vi "golpi_mpc_get_access.vi"(7 "don't query version (true)":bool=TRUE, 8 "error in":errorcluster, 10 "allow octave start (true)":bool=TRUE, 11 "golpi session ref":T1) -> (0 "error out":errorcluster, 1 "GOLPI ref out":T2={"pipe handle"={"lv_proc.dll file path"=path "", "process instance handle"=[], "debug mode"=FALSE, "debug data"=[]}, "fast read timeout [ms]"=500, "fast read settle time [ms]"=10, "fast read to multiple [ms]"=1, "max elements per input line"=100, "slow read timeout [ms]"=5000, "stdin double format specifier"="%_16e", "max elements per stdout output column"=100, "console mode bitstream"=FALSE, "bitstream first read timeout [ms]"=1000, "bitstream read timeout [ms]"=50, "struct transfer possible"=FALSE, "matlab mode"=FALSE}, 2 "golpi session out":T4={"GOLPI ref"={"pipe handle"={"lv_proc.dll file path"=path "", "process instance handle"=[], "debug mode"=FALSE, "debug data"=[]}, "fast read timeout [ms]"=500, "fast read settle time [ms]"=10, "fast read to multiple [ms]"=1, "max elements per input line"=100, "slow read timeout [ms]"=5000, "stdin double format specifier"="%_16e", "max elements per stdout output column"=100, "console mode bitstream"=FALSE, "bitstream first read timeout [ms]"=1000, "bitstream read timeout [ms]"=50, "struct transfer possible"=FALSE, "matlab mode"=FALSE}, "idn str"="", "octave path"=path "C:/Octave364/Octave3.6.4_gcc4.6.2/bin", "work path"=path "C:/Octave364/Octave3.6.4_gcc4.6.2/bin", "start timeout [ms]"=15000, "clr cache"=FALSE, "console"=FALSE, "binary"=FALSE, "semaphore"=refnum, "initial command"="", "exit command"="", "matlab"=FALSE}, 3 "golpi session ref out (copy)":T1, 4 "octave started (was closed)":bool, 5 "GNU Octave version":string)   [LabVIEW 2018, in "GOLPI Multi Process.lvlib"]
doc: "Call this to gain exclusive access to the GOLPI session (for multi-process communication). It won't return until it gets access to the GOLPI session. \n\nOptionally (by default) it will start GOLPI before returning GOLPI reference. It returns GOLPI reference - the main cluster for GOLPI library. It also returns full GOLPI session (the cluster including access semaphore and some configuarition for the mutli-process GOLPI lib). \n\nWhen work with GOLPI is done the reference must be released again by calling 'golpi_mpc_release'!"
uses:
  GOLPI Multi Process.lvlib
  golpi_session.ctl
  GOLPI Library.lvlibp/Public/GOLPI reference Type Def.ctl
  GOLPI Library.lvlibp/LV Process source distribution/Pipe Handle.ctl
  golpi_session_ref.ctl
  GOLPI Library.lvlibp/LV Process source distribution/LV Process library.lvlib
  GOLPI Library.lvlibp
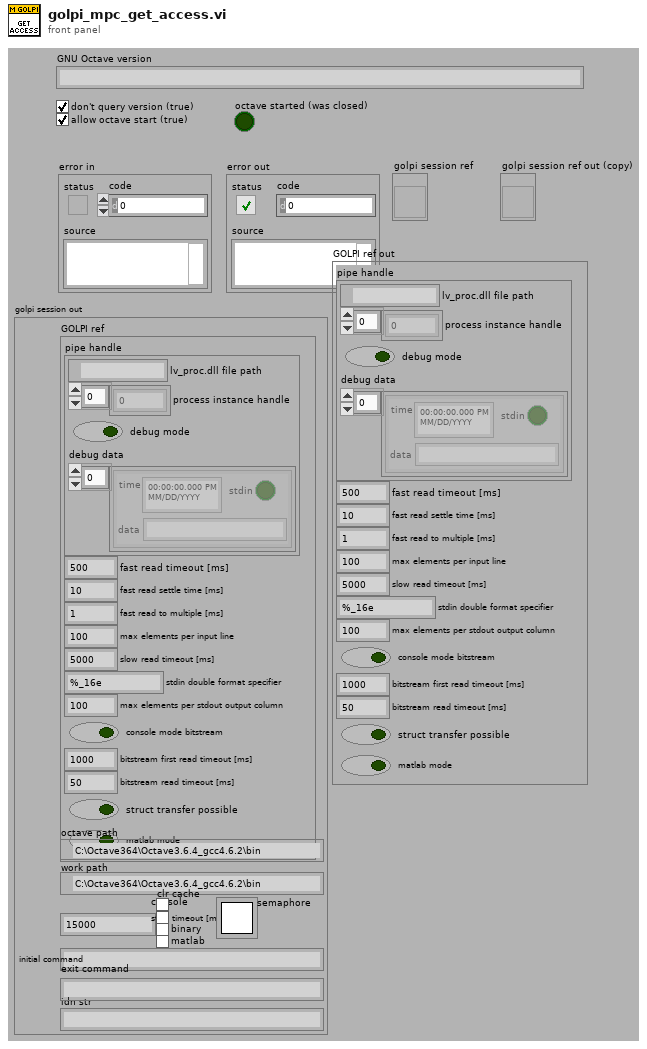
[diagram p1: front panel]
types:
  T1 = typedef "GOLPI Multi Process.lvlib/golpi_session_ref.ctl" = refnum<vi>
  T2 = typedef "GOLPI Library.lvlibp/GOLPI reference Type Def.ctl" = cluster{"pipe handle":T3, "fast read timeout [ms]":u32, "fast read settle time [ms]":u32, "fast read to multiple [ms]":u32, "max elements per input line":u32, "slow read timeout [ms]":u32, "stdin double format specifier":string, "max elements per stdout output column":u32, "console mode bitstream":bool, "bitstream first read timeout [ms]":u32, "bitstream read timeout [ms]":u32, "struct transfer possible":bool, "matlab mode":bool}
  T3 = typedef "GOLPI Library.lvlibp/LV Process library.lvlib/Pipe Handle.ctl" = cluster{"lv_proc.dll file path":path, "process instance handle":u32[], "debug mode":bool, "debug data":cluster{"time":timestamp, "stdin":bool, "data":string}[]}
  T4 = typedef "GOLPI Multi Process.lvlib/golpi_session.ctl" = cluster{"GOLPI ref":T2, "idn str":string, "octave path":path, "work path":path, "start timeout [ms]":u32, "clr cache":bool, "console":bool, "binary":bool, "semaphore":T5, "initial command":string, "exit command":string, "matlab":bool}
  T5 = typedef "Semaphore RefNum" = refnum<k1>
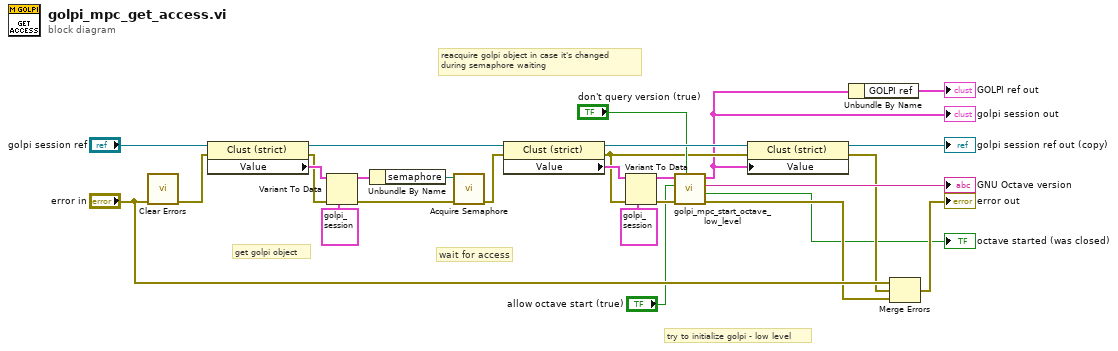
[diagram p0: block diagram]
diagram:
  # "try to initialize golpi - low level"
  # "reacquire golpi object in case it's changed\nduring semaphore waiting"
  # "wait for access"
  # "get golpi object"
  n1 = call <vilib>:"Clear Errors.vi"("error in (no error)"="error in") -> ("error out"=w12:errorcluster)  [unwired: 5 in, 1 out]
  n2 = property class="Clust (strict)"(reference="golpi session ref", error in=w12) -> (reference out=w19:T1, error out=w20:errorcluster, "Value"=w25:T4)
  n3 = Variant To Data(error in=w20, type=T4 {"GOLPI ref"={"pipe handle"={"lv_proc.dll file path"=path "", "process instance handle"=[], "debug mode"=FALSE, "debug data"=[]}, "fast read timeout [ms]"=0, "fast read settle time [ms]"=0, "fast read to multiple [ms]"=0, "max elements per input line"=0, "slow read timeout [ms]"=0, "stdin double format specifier"="", "max elements per stdout output column"=0, "console mode bitstream"=FALSE, "bitstream first read timeout [ms]"=0, "bitstream read timeout [ms]"=0, "struct transfer possible"=FALSE, "matlab mode"=FALSE}, "idn str"="", "octave path"=path "C:/Octave364/Octave3.6.4_gcc4.6.2/bin", "work path"=path "", "start timeout [ms]"=0, "clr cache"=FALSE, "console"=FALSE, "binary"=FALSE, "semaphore"=refnum, "initial command"="", "exit command"="", "matlab"=FALSE} ("golpi session"), Variant=w25) -> (data=w21:T4, error out=w23:errorcluster)
  n4 = Unbundle By Name(w21) -> ("semaphore"=w22:T5)
  n5 = call <vilib>:"Acquire Semaphore.vi"("error in (no error)"=w23, "semaphore"=w22) -> ("error out"=w16:errorcluster)  [unwired: 3 in, 2 out]
  n6 = property class="Clust (strict)"(reference=w19, error in=w16) -> (reference out=w15:T1, error out=w6:errorcluster, "Value"=w17:T4)
  n7 = Variant To Data(error in=w6, type=T4 {"GOLPI ref"={"pipe handle"={"lv_proc.dll file path"=path "", "process instance handle"=[], "debug mode"=FALSE, "debug data"=[]}, "fast read timeout [ms]"=0, "fast read settle time [ms]"=0, "fast read to multiple [ms]"=0, "max elements per input line"=0, "slow read timeout [ms]"=0, "stdin double format specifier"="", "max elements per stdout output column"=0, "console mode bitstream"=FALSE, "bitstream first read timeout [ms]"=0, "bitstream read timeout [ms]"=0, "struct transfer possible"=FALSE, "matlab mode"=FALSE}, "idn str"="", "octave path"=path "C:/Octave364/Octave3.6.4_gcc4.6.2/bin", "work path"=path "", "start timeout [ms]"=0, "clr cache"=FALSE, "console"=FALSE, "binary"=FALSE, "semaphore"=refnum, "initial command"="", "exit command"="", "matlab"=FALSE} ("golpi session"), Variant=w17) -> (data=w13:T4, error out=w14:errorcluster)
  n8 = call "golpi_mpc_start_octave_low_level.vi"("don't query version (true)"="don't query version (true)", "error in"=w14, "allow octave start (true)"="allow octave start (true)", "golpi session in"=w13) -> ("error out"=w5:errorcluster, "octave started (was closed)"=→"octave started (was closed)":bool, "GNU Octave version"=→"GNU Octave version":string, "golpi session out"=w1:T4)  [unwired: 4 in]
  "golpi session out" <- w1
  n9 = property class="Clust (strict)"(reference=w15, error in=w6, "Value"=w1) -> (reference out=→"golpi session ref out (copy)":T1, error out=w10:errorcluster)
  n10 = Unbundle By Name(w1) -> ("GOLPI ref"=→"GOLPI ref out":T2)
  n11 = Merge Errors("error in", w10, w5) -> (→"error out":errorcluster)
